vi "find targets.vi"(7 "error in":errorcluster) -> (27 "error out":errorcluster)   [LabVIEW 2011]
uses:
  <vilib>/vision/Pattern Matching.llb/IMAQ Curve Parameters.ctl
  <vilib>/vision/Pattern Matching.llb/IMAQ Match Range Setting.ctl
  <vilib>/vision/NI_Vision_Development_Module.lvlib
panel:
  out "Matches":T1(array[cluster])
  out "Image Out 4":T2(plugin-control)
  out "Image Out 3":T2(plugin-control)
  out "Image Out":T2(plugin-control)
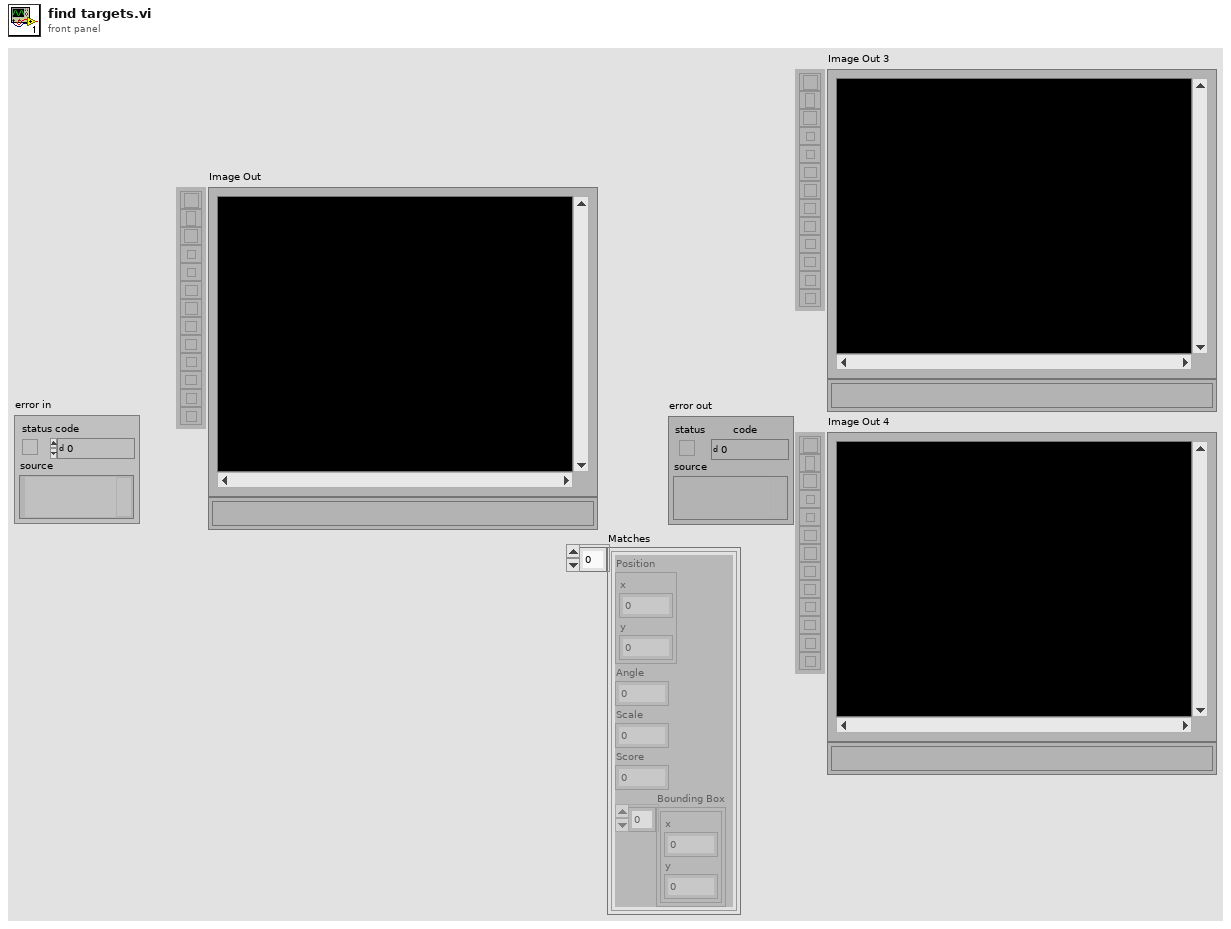
[diagram p1: front panel]
types:
  T1 = cluster{"Position":cluster{"x":sgl, "y":sgl}, "Angle":sgl, "Scale":sgl, "Score":sgl, "Bounding Box":cluster{"x":sgl, "y":sgl}[]}[]
  T2 = typedef "IMAQ Image.ctl" = refnum<image>
  T3 = cluster{"Global Rectangle":i32[], "Contours":cluster{"ID":enum32{"External", "Internal"}, "Type":u32, "Coordinates":i32[]}[]}
  T4 = typedef "IMAQ Curve Parameters.ctl" = cluster{"Extraction Mode":u32, "Edge Threshold":i32, "Edge Filter Size":u32, "Min Length":i32, "Row Search Step Size":i32, "Col Search Step Size":i32, "Max Endpoint Gap":i32, "Closed":bool, "Subpixel":bool}
  T5 = typedef "IMAQ Match Range Setting.ctl" = cluster{"Match Constraints":u32, "Min":dbl, "Max":dbl}
  T6 = cluster{"Curve Parameters":T4, "Match Mode":cluster{"Rotation":bool, "Scale":bool, "Occlusion":bool, "Reserved":bool, "Reserved":bool, "Reserved":bool}, "Range Settings":T5[], "Number of Matches":i32, "Minimum Match Score":sgl, "SubPixel Accuracy":bool, "Adv. Geometric Match Options 2":cluster{"Setup Data Item":u16, "Item Value":dbl}[]}
  T7 = typedef "Image Type" = u32
  T8 = cluster{"Match Mode":u16, "Subpixel Accuracy":bool, "Rotation Angle Ranges (degrees)":cluster{sgl, sgl}[]}
  T9 = cluster{"ROI Descriptor":cluster{"Global Rectangle":i32[], "Contours":cluster{"ID":enum32{"External", "Internal"}, "Type":u32, "Coordinates":i32[]}[]}, "Number of Matches Requested":i32, "Minimum Match Score":sgl}
  T10 = typedef "IMAQ GM Match Report.ctl" = cluster{"Position":cluster{"x":sgl, "y":sgl}, "Angle":sgl, "Scale":sgl, "Score":sgl, "Bounding Box":cluster{"x":sgl, "y":sgl}[], "Contrast Reversed":bool, "Occlusion %":sgl, "Template Target Curve Score":sgl, "Target Template Curve Score":sgl, "Correlation Score":sgl}
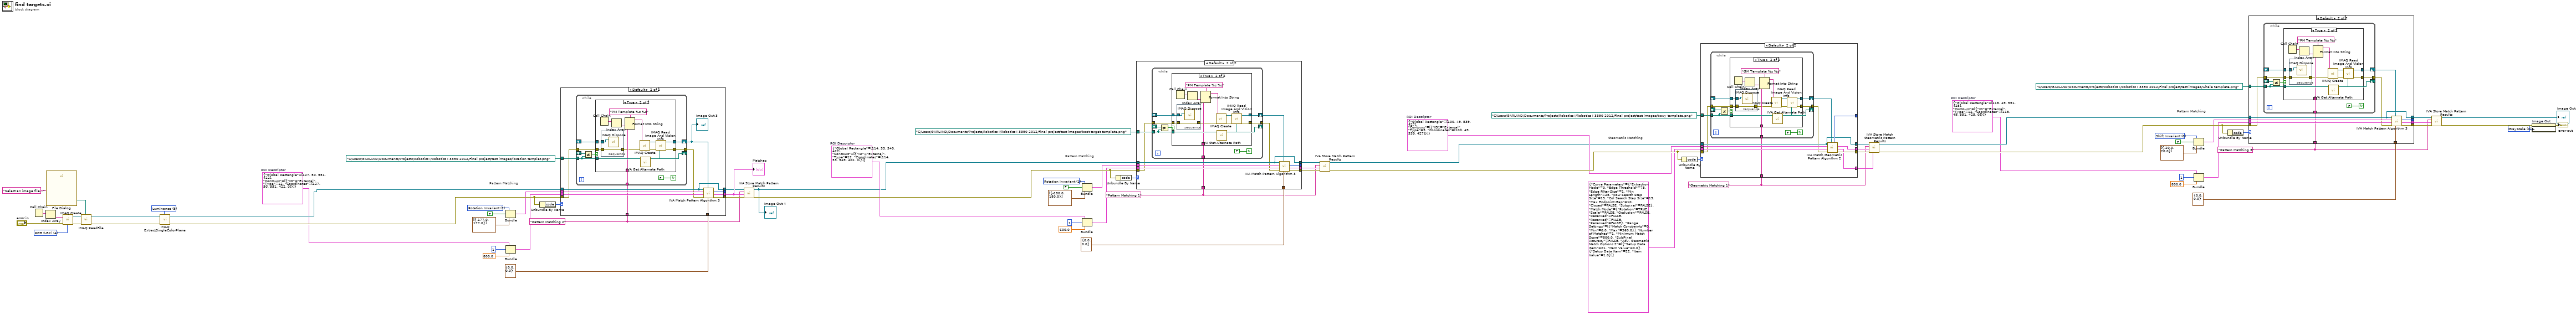
[diagram p0: block diagram]
diagram:
  w3 = u32 0 items=["Grayscale", "Binary", "Gradient", "Rainbow", "Temperature", "User Defined"] ("Palette")
  w6 = "Pattern Matching 3" ("Step Name")
  w20 = u16 0 items=["Shift Invariant", "Rotation Invariant"] ("Match Mode")
  w5 = T3 {"Global Rectangle"=[118, 49, 551, 425], "Contours"=[{"ID"=enum."External", "Type"=12, "Coordinates"=[118, 49, 551, 425, 0]}]}  # ROI Descriptor
  w22 = "Geometric Matching 1" ("Step Name")
  w31 = T3 {"Global Rectangle"=[100, 49, 539, 427], "Contours"=[{"ID"=enum."External", "Type"=3, "Coordinates"=[100, 49, 539, 427]}]}  # ROI Descriptor
  w34 = "Pattern Matching 1" ("Step Name")
  w47 = u16 1 items=["Shift Invariant", "Rotation Invariant"] ("Match Mode")
  w33 = T3 {"Global Rectangle"=[114, 53, 549, 422], "Contours"=[{"ID"=enum."External", "Type"=12, "Coordinates"=[114, 53, 549, 422, 0]}]}  # ROI Descriptor
  w50 = "Pattern Matching 2" ("Step Name")
  w64 = u16 1 items=["Shift Invariant", "Rotation Invariant"] ("Match Mode")
  w49 = T3 {"Global Rectangle"=[127, 50, 551, 422], "Contours"=[{"ID"=enum."External", "Type"=12, "Coordinates"=[127, 50, 551, 422, 0]}]}  # ROI Descriptor
  w68 = 5 items=["Red", "Green", "Blue", "Hue", "Saturation", "Luminance", "Value", "Intensity"] ("Color Plane")
  w69 = T7 4 items=["Grayscale (U8)", "Grayscale (I16)", "Grayscale (SGL)", "Complex (CSG)", "RGB (U32)", "HSL (U32)", "RGB (U64)", "Grayscale (U16)"] ("Image Type")
  # "Pattern Matching"
  # "Geometric Matching"
  # "Pattern Matching"
  # "Pattern Matching"
  n1 = Call Chain() -> (call chain=w73:string[])
  n2 = Index Array(array=w73) -> (element=w72:string)  [unwired: 1 in]
  n3 = call "File Dialog"("prompt"="Select an image file...") -> ("selected path"=w70:path)  [unwired: 6 in, 8 out]
  n4 = call "IMAQ Create"("Image Name"=w72, "Image Type"=w69, "error in (no error)"="error in") -> ("New Image"=w76:T2, "error out"=w75:errorcluster)  [unwired: 1 in, 1 out]
  n5 = call "IMAQ ReadFile"("File Path"=w70, "error in (no error)"=w75, "Image"=w76) -> ("error out"=w77:errorcluster, "Image Out"=w67:T2)  [unwired: 2 in, 5 out]
  n6 = call "IMAQ ExtractSingleColorPlane"("Color Plane"=w68, "error in (no error)"=w77, "Image Src"=w67) -> ("error out"=w66:errorcluster, "Image Dst Out"=w56:T2)  [unwired: 1 in, 6 out]
  n7 = Bundle("Match Mode"=w64, "Subpixel Accuracy"=FALSE, "Rotation Angle Ranges (degrees)"=cluster{sgl, sgl}[] [{-177.0, 177.0}]) -> (w61:T8)  [unwired: 1 out]
  n8 = Bundle("ROI Descriptor"=w49, "Number of Matches Requested"=1, "Minimum Match Score"=sgl 800.0) -> (w58:T9)  [unwired: 1 out]
  n9 = Unbundle By Name(w66) -> ("code"=w51:i32)
  n10 = case shown="Default" w51 {
    tunnel: path "C:/Users/GARLAND/Documents/Projects/Robotics I/Robotics I 3390 2012/Final project/test images/location templet.png" ("Template File Path") -> [_ w83]
    tunnel: w66 -> [_ w82]
    tunnel: [_ w90] -> _
    tunnel: w61 -> [_ w89]
    tunnel: w58 -> [_ w88]
    tunnel: cluster{"X":sgl, "Y":sgl} {"X"=0.0, "Y"=0.0} ("Match Offset") -> [_ w87]
    tunnel: w56 -> [w78 w84]
    tunnel: [_ w86] -> w55
    tunnel: [_ w85] -> w53
    tunnel: [w78 w84] -> w52
    tunnel: w50 -> [_ w80]
    frame -1074396199, -1074396198 {
      # "Discard\nCoordinate\nSystem Error"
    }
    frame Default {
      n11 = while {
        shift-right: [w99] -> w79
        shift-left: _ -> [w98]
        tunnel: [w96] -> w81
        tunnel: w82 -> [w95]
        tunnel: w83 -> [w92]
        tunnel: w80 -> [w94]
        shift-right: [w92] -> _
        shift-left: _ -> [w93]
        stop <- FALSE continue-if-true
        n12 = Not Equal?(x=w93, y=w92) -> (x != y?=w91:bool)
        n13 = case shown="True" w91 {
          tunnel: [w101 w113] -> w99
          tunnel: w98 -> [w101 w104]
          tunnel: [w100 w110] -> w96
          tunnel: w95 -> [w100 w103]
          tunnel: w92 -> [_ w106]
          tunnel: w94 -> [_ w107]
          frame False {
          }
          frame True {
            n14 = Call Chain() -> (call chain=w109:string[])
            n15 = stacked-sequence {
              tunnel: w104 -> [w117]
              tunnel: w103 -> [w116]
              tunnel: [w116] -> w102
              frame #0 {
                n16 = call "IMAQ Dispose"("Image"=w117) -> ()  [unwired: 2 in, 4 out]
              }
            }
            n17 = Index Array(array=w109) -> (element=w108:string)  [unwired: 1 in]
            n18 = Format Into String(format string="PM Template %s %s" ("Image Name"), w108, w107) -> (resulting string=w115:string)  [unwired: 2 in, 1 out]
            n19 = call "IMAQ Create"("Image Name"=w115, "error in (no error)"=w102) -> ("New Image"=w112:T2, "error out"=w111:errorcluster)  [unwired: 2 in, 1 out]
            n20 = call <vilib>:"IVA Get Alternate Path.vi"("Path In"=w106) -> ("Path Out"=w105:path)  [unwired: 10 out]
            n21 = call "IMAQ Read Image And Vision Info"("File Path"=w105, "error in (no error)"=w111, "Image"=w112) -> ("error out"=w110:errorcluster, "Image Out"=w113:T2)  [unwired: 1 in, 6 out]
          }
        }
      }
      "Image Out 3" <- w79
      n22 = call <vilib>:"IVA Match Pattern Algorithm 3.vi"("Match Offset"=w87, "Image Template"=w79, "error in (no error)"=w81, "Match Parameters"=w88, "Setup Match Parameters"=w89, "Image"=w84) -> ("error out"=w86:errorcluster, "Number of Matches"=w90:i32, "Matches"=w85:T1)  [unwired: 3 out]
    }
  }
  "Matches" <- w53
  n23 = call <vilib>:"IVA Store Match Pattern Results.vi"("error in (no error)"=w55, "Matches"=w53, "Step Name"=w50, "Image in"=w52) -> ("error out"=w54:errorcluster, "Image dup"=w1:T2)  [unwired: 6 out]
  "Image Out 4" <- w1
  n24 = Bundle("Match Mode"=w47, "Subpixel Accuracy"=FALSE, "Rotation Angle Ranges (degrees)"=cluster{sgl, sgl}[] [{-180.0, 180.0}]) -> (w44:T8)  [unwired: 1 out]
  n25 = Bundle("ROI Descriptor"=w33, "Number of Matches Requested"=1, "Minimum Match Score"=sgl 600.0) -> (w41:T9)  [unwired: 1 out]
  n26 = Unbundle By Name(w54) -> ("code"=w35:i32)
  n27 = case shown="Default" w35 {
    tunnel: path "C:/Users/GARLAND/Documents/Projects/Robotics I/Robotics I 3390 2012/Final project/test images/boat target templete.png" ("Template File Path") -> [_ w123]
    tunnel: w54 -> [_ w122]
    tunnel: [_ w130] -> _
    tunnel: w44 -> [_ w129]
    tunnel: w41 -> [_ w128]
    tunnel: cluster{"X":sgl, "Y":sgl} {"X"=0.0, "Y"=0.0} ("Match Offset") -> [_ w127]
    tunnel: w1 -> [w118 w124]
    tunnel: [_ w126] -> w39
    tunnel: [_ w125] -> w37
    tunnel: [w118 w124] -> w36
    tunnel: w34 -> [_ w119]
    frame -1074396199, -1074396198 {
      # "Discard\nCoordinate\nSystem Error"
    }
    frame Default {
      n28 = while {
        shift-right: [w139] -> w120
        shift-left: _ -> [w138]
        tunnel: [w136] -> w121
        tunnel: w122 -> [w135]
        tunnel: w123 -> [w132]
        tunnel: w119 -> [w134]
        shift-right: [w132] -> _
        shift-left: _ -> [w133]
        stop <- FALSE continue-if-true
        n29 = Not Equal?(x=w133, y=w132) -> (x != y?=w131:bool)
        n30 = case shown="True" w131 {
          tunnel: [w141 w153] -> w139
          tunnel: w138 -> [w141 w144]
          tunnel: [w140 w150] -> w136
          tunnel: w135 -> [w140 w143]
          tunnel: w132 -> [_ w146]
          tunnel: w134 -> [_ w147]
          frame False {
          }
          frame True {
            n31 = Call Chain() -> (call chain=w149:string[])
            n32 = stacked-sequence {
              tunnel: w144 -> [w157]
              tunnel: w143 -> [w156]
              tunnel: [w156] -> w142
              frame #0 {
                n33 = call "IMAQ Dispose"("Image"=w157) -> ()  [unwired: 2 in, 4 out]
              }
            }
            n34 = Index Array(array=w149) -> (element=w148:string)  [unwired: 1 in]
            n35 = Format Into String(format string="PM Template %s %s" ("Image Name"), w148, w147) -> (resulting string=w155:string)  [unwired: 2 in, 1 out]
            n36 = call "IMAQ Create"("Image Name"=w155, "error in (no error)"=w142) -> ("New Image"=w152:T2, "error out"=w151:errorcluster)  [unwired: 2 in, 1 out]
            n37 = call <vilib>:"IVA Get Alternate Path.vi"("Path In"=w146) -> ("Path Out"=w145:path)  [unwired: 10 out]
            n38 = call "IMAQ Read Image And Vision Info"("File Path"=w145, "error in (no error)"=w151, "Image"=w152) -> ("error out"=w150:errorcluster, "Image Out"=w153:T2)  [unwired: 1 in, 6 out]
          }
        }
      }
      n39 = call <vilib>:"IVA Match Pattern Algorithm 3.vi"("Match Offset"=w127, "Image Template"=w120, "error in (no error)"=w121, "Match Parameters"=w128, "Setup Match Parameters"=w129, "Image"=w124) -> ("error out"=w126:errorcluster, "Number of Matches"=w130:i32, "Matches"=w125:T1)  [unwired: 3 out]
    }
  }
  n40 = call <vilib>:"IVA Store Match Pattern Results.vi"("error in (no error)"=w39, "Matches"=w37, "Step Name"=w34, "Image in"=w36) -> ("error out"=w38:errorcluster, "Image dup"=w30:T2)  [unwired: 6 out]
  n41 = Unbundle By Name(w38) -> ("code"=w25:i32)
  n42 = case shown="Default" w25 {
    tunnel: path "C:/Users/GARLAND/Documents/Projects/Robotics I/Robotics I 3390 2012/Final project/test images/bouy templete.png" ("Template File Path") -> [_ w163]
    tunnel: w38 -> [_ w162]
    tunnel: T6 {"Curve Parameters"={"Extraction Mode"=0, "Edge Threshold"=75, "Edge Filter Size"=1, "Min Length"=25, "Row Search Step Size"=15, "Col Search Step Size"=15, "Max Endpoint Gap"=10, "Closed"=FALSE, "Subpixel"=FALSE}, "Match Mode"={"Rotation"=TRUE, "Scale"=FALSE, "Occlusion"=FALSE, "Reserved"=FALSE, "Reserved"=FALSE, "Reserved"=FALSE}, "Range Settings"=[{"Match Constraints"=0, "Min"=0.0, "Max"=360.0}], "Number of Matches"=1, "Minimum Match Score"=800.0, "SubPixel Accuracy"=FALSE, "Adv. Geometric Match Options 2"=[{"Setup Data Item"=21, "Item Value"=0.0}, {"Setup Data Item"=22, "Item Value"=1.0}]} ("Settings") -> [_ w170]
    tunnel: w31 -> [_ w169]
    tunnel: w30 -> [w158 w164]
    tunnel: [_ w168] -> w29
    tunnel: [_ w167] -> w27
    tunnel: [_ w166] -> w26
    tunnel: [_ w165] -> _
    tunnel: [w158 w164] -> w24
    tunnel: w22 -> [_ w159]
    frame -1074396199, -1074396198 {
      # "Discard Coordinate System Error"
    }
    frame Default {
      n43 = while {
        shift-right: [w179] -> w160
        shift-left: _ -> [w178]
        tunnel: [w176] -> w161
        tunnel: w162 -> [w175]
        tunnel: w163 -> [w171]
        tunnel: w159 -> [w174]
        shift-right: [w171] -> _
        shift-left: _ -> [w173]
        stop <- FALSE continue-if-true
        n44 = Not Equal?(x=w173, y=w171) -> (x != y?=w172:bool)
        n45 = case shown="True" w172 {
          tunnel: [w181 w193] -> w179
          tunnel: w178 -> [w181 w185]
          tunnel: [w180 w190] -> w176
          tunnel: w175 -> [w180 w186]
          tunnel: w174 -> [_ w187]
          tunnel: w171 -> [_ w183]
          frame False {
          }
          frame True {
            n46 = Call Chain() -> (call chain=w189:string[])
            n47 = stacked-sequence {
              tunnel: w186 -> [w197]
              tunnel: w185 -> [w196]
              tunnel: [w197] -> w184
              frame #0 {
                n48 = call "IMAQ Dispose"("Image"=w196) -> ()  [unwired: 2 in, 4 out]
              }
            }
            n49 = Index Array(array=w189) -> (element=w188:string)  [unwired: 1 in]
            n50 = Format Into String(format string="GM Template %s %s" ("Image Name"), w188, w187) -> (resulting string=w195:string)  [unwired: 2 in, 1 out]
            n51 = call "IMAQ Create"("Image Name"=w195, "error in (no error)"=w184) -> ("New Image"=w192:T2, "error out"=w191:errorcluster)  [unwired: 2 in, 1 out]
            n52 = call <vilib>:"IVA Get Alternate Path.vi"("Path In"=w183) -> ("Path Out"=w182:path)  [unwired: 10 out]
            n53 = call "IMAQ Read Image And Vision Info"("File Path"=w182, "error in (no error)"=w191, "Image"=w192) -> ("error out"=w190:errorcluster, "Image Out"=w193:T2)  [unwired: 1 in, 6 out]
          }
        }
      }
      n54 = call <vilib>:"IVA Match Geometric Pattern Algorithm 2.vi"("Template"=w160, "error in (no error)"=w161, "Settings"=w170, "ROI Descriptor"=w169, "Image"=w164) -> ("error out"=w168:errorcluster, "Calibrated Matches"=w166:T10[], "Matches"=w167:T10[], "Number of Matches"=w165:i32)  [unwired: 1 in, 2 out]
    }
  }
  n55 = call <vilib>:"IVA Store Match Geometric Pattern Results.vi"("Calibrated Matches"=w26, "error in (no error)"=w29, "Matches"=w27, "Step Name"=w22, "Image in"=w24) -> ("error out"=w28:errorcluster, "Image dup"=w12:T2)  [unwired: 5 out]
  n56 = Bundle("Match Mode"=w20, "Subpixel Accuracy"=FALSE, "Rotation Angle Ranges (degrees)"=cluster{sgl, sgl}[] [{-20.0, 20.0}]) -> (w17:T8)  [unwired: 1 out]
  n57 = Bundle("ROI Descriptor"=w5, "Number of Matches Requested"=1, "Minimum Match Score"=sgl 800.0) -> (w14:T9)  [unwired: 1 out]
  n58 = Unbundle By Name(w28) -> ("code"=w7:i32)
  n59 = case shown="Default" w7 {
    tunnel: path "C:/Users/GARLAND/Documents/Projects/Robotics I/Robotics I 3390 2012/Final project/test images/whale templete.png" ("Template File Path") -> [_ w203]
    tunnel: w28 -> [_ w202]
    tunnel: [_ w210] -> _
    tunnel: w17 -> [_ w209]
    tunnel: w14 -> [_ w208]
    tunnel: cluster{"X":sgl, "Y":sgl} {"X"=0.0, "Y"=0.0} ("Match Offset") -> [_ w207]
    tunnel: w12 -> [w198 w204]
    tunnel: [_ w206] -> w11
    tunnel: [_ w205] -> w9
    tunnel: [w198 w204] -> w8
    tunnel: w6 -> [_ w199]
    frame -1074396199, -1074396198 {
      # "Discard\nCoordinate\nSystem Error"
    }
    frame Default {
      n60 = while {
        shift-right: [w219] -> w200
        shift-left: _ -> [w218]
        tunnel: [w216] -> w201
        tunnel: w202 -> [w215]
        tunnel: w203 -> [w212]
        tunnel: w199 -> [w214]
        shift-right: [w212] -> _
        shift-left: _ -> [w213]
        stop <- FALSE continue-if-true
        n61 = Not Equal?(x=w213, y=w212) -> (x != y?=w211:bool)
        n62 = case shown="True" w211 {
          tunnel: [w221 w233] -> w219
          tunnel: w218 -> [w221 w224]
          tunnel: [w220 w230] -> w216
          tunnel: w215 -> [w220 w223]
          tunnel: w212 -> [_ w226]
          tunnel: w214 -> [_ w227]
          frame False {
          }
          frame True {
            n63 = Call Chain() -> (call chain=w229:string[])
            n64 = stacked-sequence {
              tunnel: w224 -> [w237]
              tunnel: w223 -> [w236]
              tunnel: [w236] -> w222
              frame #0 {
                n65 = call "IMAQ Dispose"("Image"=w237) -> ()  [unwired: 2 in, 4 out]
              }
            }
            n66 = Index Array(array=w229) -> (element=w228:string)  [unwired: 1 in]
            n67 = Format Into String(format string="PM Template %s %s" ("Image Name"), w228, w227) -> (resulting string=w235:string)  [unwired: 2 in, 1 out]
            n68 = call "IMAQ Create"("Image Name"=w235, "error in (no error)"=w222) -> ("New Image"=w232:T2, "error out"=w231:errorcluster)  [unwired: 2 in, 1 out]
            n69 = call <vilib>:"IVA Get Alternate Path.vi"("Path In"=w226) -> ("Path Out"=w225:path)  [unwired: 10 out]
            n70 = call "IMAQ Read Image And Vision Info"("File Path"=w225, "error in (no error)"=w231, "Image"=w232) -> ("error out"=w230:errorcluster, "Image Out"=w233:T2)  [unwired: 1 in, 6 out]
          }
        }
      }
      n71 = call <vilib>:"IVA Match Pattern Algorithm 3.vi"("Match Offset"=w207, "Image Template"=w200, "error in (no error)"=w201, "Match Parameters"=w208, "Setup Match Parameters"=w209, "Image"=w204) -> ("error out"=w206:errorcluster, "Number of Matches"=w210:i32, "Matches"=w205:T1)  [unwired: 3 out]
    }
  }
  n72 = call <vilib>:"IVA Store Match Pattern Results.vi"("error in (no error)"=w11, "Matches"=w9, "Step Name"=w6, "Image in"=w8) -> ("error out"=w10:errorcluster, "Image dup"=→"Image Out":T2)  [unwired: 6 out]
  n73 = property on="Image Out" class="ImageControl"(error in=w10, "Palette:Palette Type"=w3) -> (error out=→"error out":errorcluster)  [unwired: 1 in, 1 out]
